vi "Actor Core.vi"(8 "error in":errorcluster, 11 "RDS Router Actor in":refnum<class "RDS Router Actor.lvclass">) -> (0 "error out":errorcluster, 3 "Actor out":refnum<class "Actor.lvclass">)   [LabVIEW 2015]
doc: "(<B>Filename</B>: Actor Framework.lvlib:Actor.lvclass:Actor Core.vi)\n\nReceives messages to the actor, reacts to them, and initiates any error handling that may shut the actor down.\n\nDescendant classes may override this VI to append parallel tasks for the actor to complete while it handles messages. Overrides use the Call Parent Method node."
uses:
  <vilib>/ActorFramework/Actor/Actor.lvclass
  RDS Router Actor.lvclass
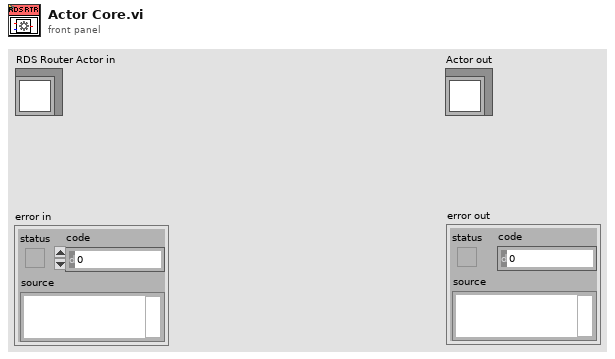
[diagram p1: front panel]
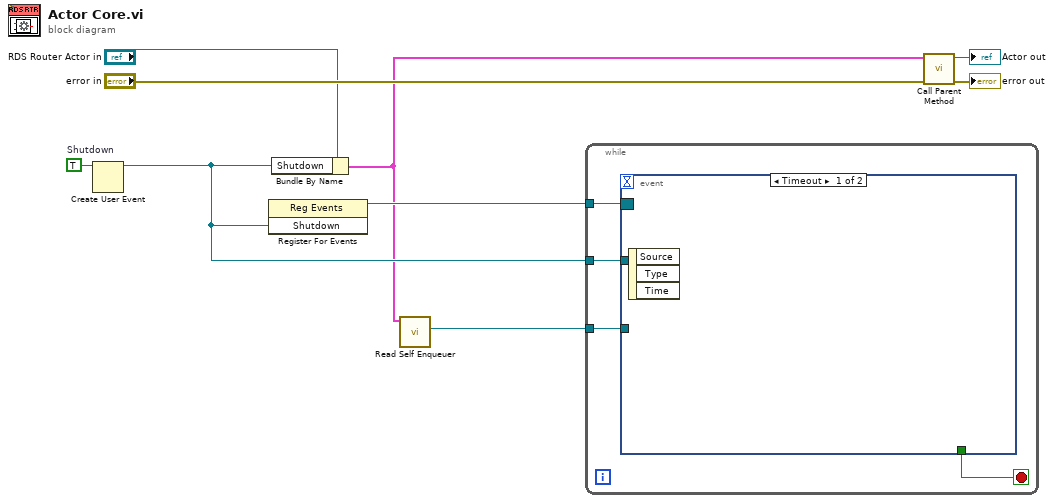
[diagram p0: block diagram]
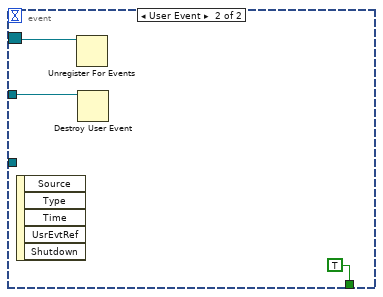
[diagram p2: hidden frame]
diagram:
  w5 = TRUE  # Shutdown
  n1 = Create User Event(user event datatype=w5) -> (user event=w3:refnum<user-event>)  [unwired: 1 in, 1 out]
  n2 = register-events(w3) -> (reference out=w4:refnum<event-registration>)  [unwired: 2 in, 1 out]
  n3 = Bundle By Name(cluster="RDS Router Actor in", "Shutdown"=w3) -> (w1:cluster{})
  n4 = call <vilib>:"Read Self Enqueuer.vi"("Actor"=w1) -> ("Self Enqueuer"=w6:refnum<class "Message Enqueuer.lvclass">)  [unwired: 10 in]
  n5 = while {
    tunnel: w6 -> [w13]
    tunnel: w4 -> [w12]
    tunnel: w3 -> [w10]
    stop <- w11 stop-if-true
    n6 = event shown="[0] Timeout" {
      selector: w12 -> [_ w15]
      dyn-events: _ -> [_ _]
      timeout: _ -> [_ _]
      tunnel: w13 -> [_ _]
      tunnel: [_ TRUE] -> w11
      tunnel: w10 -> [_ w14]
      event Timeout {
        n7 = event-data() -> ()  [unwired: 1 in, 3 out]
      }
      event User Event {
        n8 = event-data() -> ()  [unwired: 1 in, 5 out]
        n9 = Unregister For Events(event registration refnum=w15) -> ()  [unwired: 1 in, 1 out]
        n10 = Destroy User Event(user event=w14) -> ()  [unwired: 1 in, 1 out]
      }
    }
  }
  n11 = call-parent "Call Parent Method"("error in"="error in", "Actor in"=w1) -> ("error out"=→"error out":errorcluster, "Actor out"=→"Actor out":refnum<class "Actor.lvclass">)  [unwired: 8 in]
